vi "Mathematical Morphological Filter.vi"(7 "X extension type":u16(ring) items=["Zero padding", "Symmetric", "Periodic"], 8 "zero phase?":bool=TRUE, 9 "operation type":u16(ring) items=["Dilation", "Erosion"], 10 "Structure Element":dbl[](array[numeric]), 11 "X":dbl[](array[numeric])) -> (0 "error":i32, 3 "Filtered X":dbl[](array[numeric]))   [LabVIEW 2017, in "NI_AAL_Filter.lvlib"]
doc: "Filters the input data sequence <B>X</B> with <B>Structure Element</B> using a mathematical morphological filter."
uses:
  <vilib>/Analysis/NI_AAL_Filter.lvlib
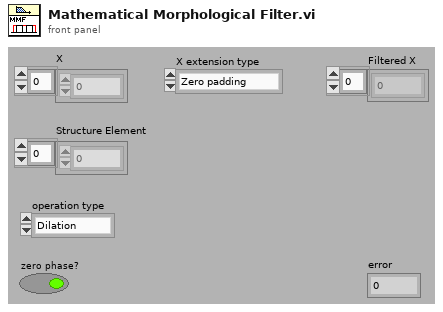
[diagram p1: front panel]
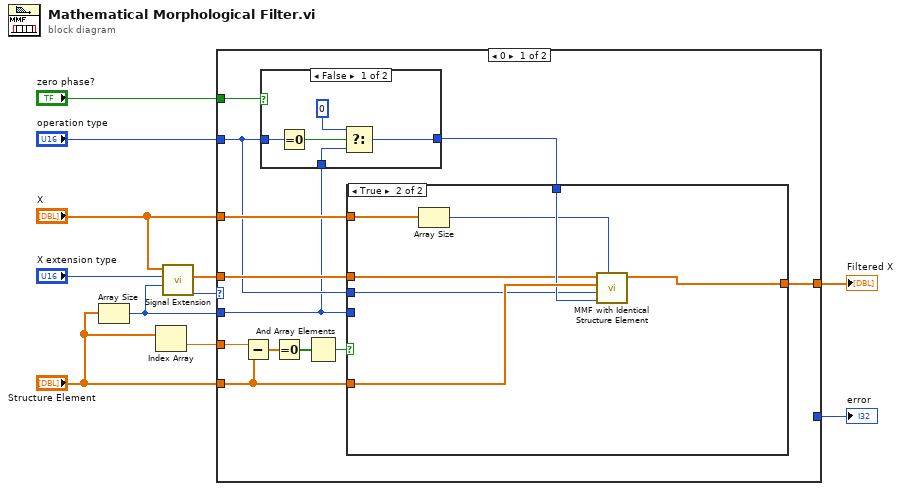
[diagram p0: block diagram]
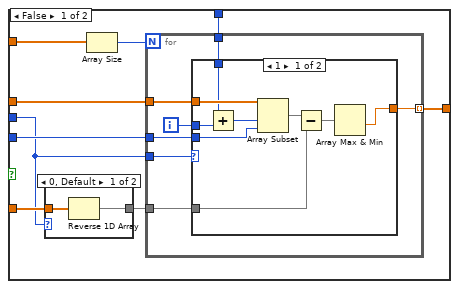
[diagram p2: hidden frame]
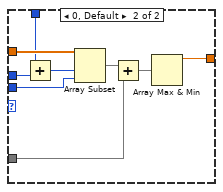
[diagram p4: hidden frame]
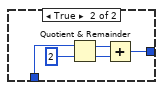
[diagram p5: hidden frame]
diagram:
  n1 = Array Size(array="Structure Element") -> (size(s)=w5:i32)
  n2 = Index Array(array="Structure Element") -> (element=w1:dbl)  [unwired: 1 in]
  n3 = call <vilib>:"Signal Extension.vi"("extension length"=w5, "X extension type"="X extension type", "X In"="X") -> ("error"=w4:i32, "X Out"=w11:dbl[])  [unwired: 5 in, 2 out]
  n4 = case shown="0" w4 {
    selector: w4 -> [_ w78]
    tunnel: w11 -> [w23 _]
    tunnel: "X" -> [w22 _]
    tunnel: [w21 _] -> w9
    tunnel: "zero phase?" -> [w15 _]
    tunnel: "operation type" -> [w14 _]
    tunnel: w5 -> [w13 _]
    tunnel: "Structure Element" -> [w18 _]
    tunnel: [_ w78] -> w3
    tunnel: w1 -> [w16 _]
    frame 0 {
      n5 = Subtract(x=w16, y=w18) -> (x-y=w19:dbl[])
      n6 = case shown="False" w15 {
        tunnel: w14 -> [w72 _]
        tunnel: w13 -> [w69 w77]
        tunnel: [w68 w73] -> w12
        frame False {
          n7 = Equal To 0?(x=w72) -> (x = 0?=w71:bool)
          n8 = Select(t=0, s=w71, f=w69) -> (s? t:f=w68:i32)
        }
        frame True {
          n9 = Quotient & Remainder(x=w77, y=2) -> (x-y*floor(x/y)=w74:i32, floor(x/y)=w75:i32)
          n10 = Add(x=w74, y=w75) -> (x+y=w73:i32)
        }
      }
      n11 = Equal To 0?(x=w19) -> (x = 0?=w20:bool[])
      n12 = And Array Elements(Boolean array=w20) -> (logical AND=w17:bool)
      n13 = case shown="True" w17 {
        tunnel: w23 -> [w32 w63]
        tunnel: w22 -> [w31 w62]
        tunnel: [w29 w65] -> w21
        tunnel: w13 -> [w27 _]
        tunnel: w18 -> [w26 w67]
        tunnel: w14 -> [w25 w64]
        tunnel: w12 -> [w24 w66]
        frame False {
          n14 = case shown="0, Default" w25 {
            tunnel: w26 -> [w34 w35]
            tunnel: [w33 w35] -> w28
            frame 0, Default {
              n15 = Reverse 1D Array(array=w34) -> (reversed array=w33:dbl[])
            }
            frame 1 {
            }
          }
          n16 = Array Size(array=w31) -> (size(s)=w30:i32)
          n17 = for {
            N: w30 -> [_]
            tunnel: w32 -> [w40]
            tunnel: w27 -> [w41]
            tunnel: w25 -> [w42]
            tunnel: [w39] -> w29 mode=indexing
            tunnel: w28 -> [w38]
            tunnel: w24 -> [w36]
            i -> [w37]
            n18 = case shown="1" w42 {
              tunnel: w41 -> [w46 w59]
              tunnel: w40 -> [w51 w60]
              tunnel: [w50 w58] -> w39
              tunnel: w37 -> [w44 w52]
              tunnel: w38 -> [w47 w55]
              tunnel: w36 -> [w43 w53]
              frame 1 {
                n19 = Add(x=w43, y=w44) -> (x+y=w45:i32)
                n20 = Array Subset(array=w51, index=w45, length=w46) -> (w49:dbl[])
                n21 = Subtract(x=w49, y=w47) -> (x-y=w48:dbl[])
                n22 = Array Max & Min(array=w48) -> (min value=w50:dbl)  [unwired: 3 out]
              }
              frame 0, Default {
                n23 = Add(x=w53, y=w52) -> (x+y=w54:i32)
                n24 = Array Subset(array=w60, index=w54, length=w59) -> (w56:dbl[])
                n25 = Add(x=w56, y=w55) -> (x+y=w57:dbl[])
                n26 = Array Max & Min(array=w57) -> (max value=w58:dbl)  [unwired: 3 out]
              }
            }
          }
        }
        frame True {
          n27 = Array Size(array=w62) -> (size(s)=w61:i32)
          n28 = call <vilib>:"MMF with Identical Structure Element.vi"("signal length"=w61, "start index"=w66, "operation type"=w64, "Structure Element"=w67, "Extended X"=w63) -> ("Filtered X"=w65:dbl[])  [unwired: 6 in]
        }
      }
    }
    frame 1, Default {
    }
  }
  "Filtered X" <- w9
  "error" <- w3
